vi "Build Command String.vi"(1 "Executable":string, 2 "Arguments":string) -> (0 "Command String":string)   [LabVIEW 2020, in "serenial.io-ase.lvlib" / "ase.lvclass"]
uses:
  ase.lvclass
  ase.lvclass/ase.ctl
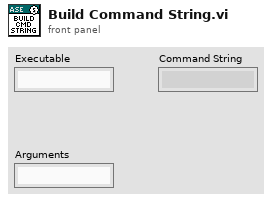
[diagram p1: front panel]
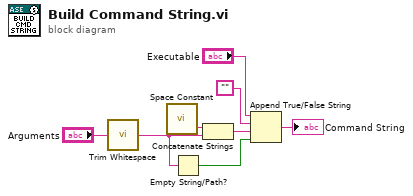
[diagram p0: block diagram]
diagram:
  n1 = call "Trim Whitespace.vi"("Input"="Arguments") -> ("Output"=w1:string)
  n2 = call <vilib>:"Space Constant.vi"() -> ("String"=w4:string)
  n3 = Empty String/Path?(string/path=w1) -> (empty?=w3:bool)
  n4 = Concatenate Strings(w4, w1) -> (w5:string)
  n5 = Append True/False String(1:w3, 2:w5, 3:"", 4:"Executable") -> (0:→"Command String":string)
